vi "rs3 showError.vi"(8 "error in (no error)":errorcluster, 11 "error":u64) -> (0 "error out":errorcluster, 1 "error message":string, 2 "Failed args":string, 3 "Failed Function":string, 5 "Error summary":string)   [LabVIEW 2017, in "libRealSense3.lvlib"]
doc: "Describes the Error received from any any previous libRealSense VI"
uses:
  <vilib>/addons/RealSense/libRealSense3.lvlib
panel:
  # "RS3 Show Errors"
  # "(C) Intel Corp.,  AGJ"
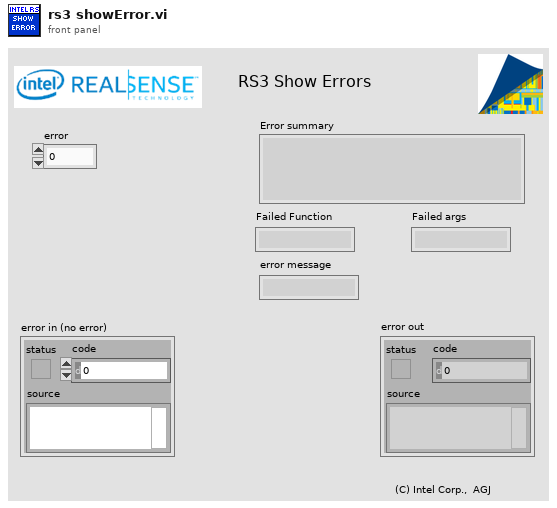
[diagram p1: front panel]
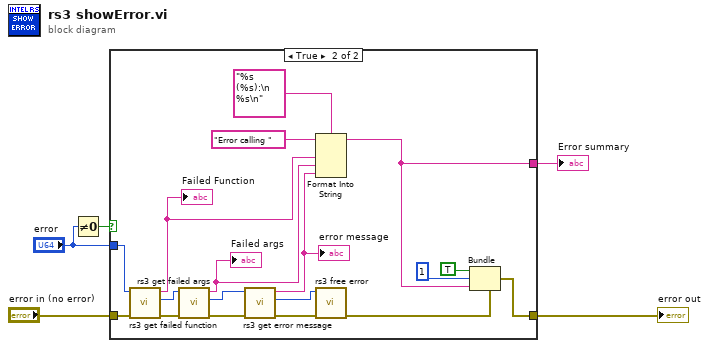
[diagram p0: block diagram]
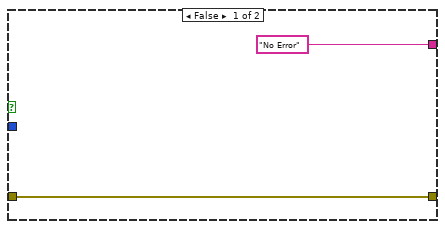
[diagram p2: hidden frame]
diagram:
  n1 = Not Equal To 0?(x="error") -> (x != 0?=w2:bool)
  n2 = case shown="True" w2 {
    tunnel: "error in (no error)" -> [w7 w25]
    tunnel: [w7 w11] -> w4
    tunnel: "error" -> [_ w23]
    tunnel: ["No Error" w10] -> w3
    frame False {
    }
    frame True {
      n3 = call <vilib>:"rs3 get failed function.vi"("error in (no error)"=w25, "error in"=w23) -> (0:"error out"=w13:errorcluster, 2:"error out"=w16:u64, "Failed Function"=w20:string)  [unwired: 7 in]
      "Failed Function" <- w20
      n4 = call <vilib>:"rs3 get failed args.vi"("error in (no error)"=w13, "error in"=w16) -> (0:"error out"=w14:errorcluster, 2:"error out"=w17:u64, "Failed args"=w21:string)  [unwired: 7 in]
      "Failed args" <- w21
      n5 = call <vilib>:"rs3 get error message.vi"("error in (no error)"=w14, "error in"=w17) -> (0:"error out"=w15:errorcluster, 2:"error out"=w24:u64, "error message"=w22:string)  [unwired: 7 in]
      "error message" <- w22
      n6 = Format Into String(format string="%s (%s):\n %s\n", initial string="Error calling ", w20, w21, w22) -> (resulting string=w10:string)  [unwired: 1 in, 1 out]
      n7 = call <vilib>:"rs3 free error.vi"("error in (no error)"=w15, "error in"=w24) -> ("error out 2"=w12:errorcluster)  [unwired: 8 in, 1 out]
      n8 = Bundle(cluster=w12, "status"=TRUE, "code"=1, "source"=w10) -> (w11:errorcluster)
    }
  }
  "Error summary" <- w3
  "error out" <- w4
